vi "Disconnect.vi"(8 "error in":errorcluster, 11 "5105 in":refnum<class "5105.lvclass">) -> (0 "error out":errorcluster, 3 "5105 out":refnum<class "5105.lvclass">)   [LabVIEW 2019, in "5105.lvlib" / "5105.lvclass"]
uses:
  5105.lvclass
  Accessors/Read Local Resource.vi
  Accessors/Write Local Resource.vi
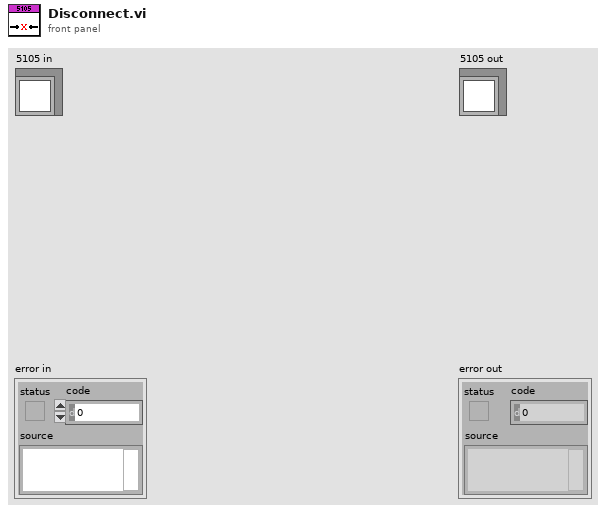
[diagram p1: front panel]
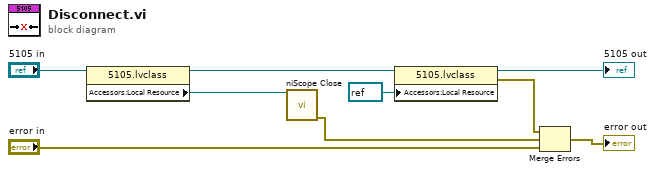
[diagram p0: block diagram]
diagram:
  n1 = property class="5105.lvclass"(reference="5105 in") -> (reference out=w5:refnum<class "5105.lvclass">, "Accessors:Local Resource"=w6:refnum<k15>)  [unwired: 1 in, 1 out]
  n2 = call <instrlib>:"niScope Close.vi"("instrument handle"=w6) -> ("error out"=w3:errorcluster)  [unwired: 14 in]
  n3 = property class="5105.lvclass"(reference=w5, "Accessors:Local Resource"=refnum<k15> refnum ("Local Resource")) -> (reference out=→"5105 out":refnum<class "5105.lvclass">, error out=w1:errorcluster)  [unwired: 1 in]
  n4 = Merge Errors(w1, w3, "error in") -> (→"error out":errorcluster)
